vi "Read XML_Extra Checks.vi"(8 "error in (no error)":errorcluster, 11 "Channels In":T1[](array[typedef])) -> (0 "error out":errorcluster, 3 "Channels Out":T1[](array[typedef]))   [LabVIEW 2020]
doc: "This VI performs extra checks (to what is done via the XML Deserializer with the XSD)."
uses:
  XML_Channel.ctl
  XML_Label.ctl
  XML_Parameter.ctl
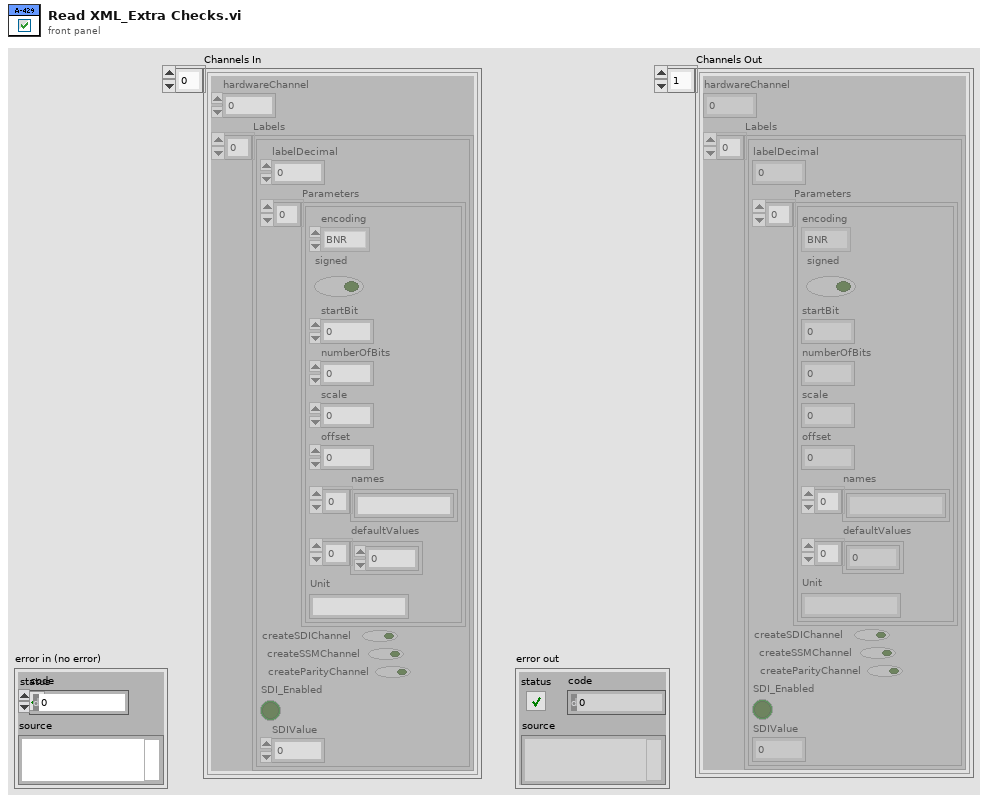
[diagram p1: front panel]
types:
  T1 = typedef "XML_Channel.ctl" = cluster{"hardwareChannel":i32, "Labels":T2[]}
  T2 = typedef "XML_Label.ctl" = cluster{"labelDecimal":i32, "Parameters":T3[], "createSDIChannel":bool, "createSSMChannel":bool, "createParityChannel":bool, "SDI_Enabled":bool, "SDIValue":u8}
  T3 = typedef "XML_Parameter.ctl" = cluster{"encoding":enum16{"BNR", "BCD", "Discrete"}, "signed":bool, "startBit":i32, "numberOfBits":i32, "scale":dbl, "offset":dbl, "names":string[], "defaultValues":dbl[], "Unit":string}
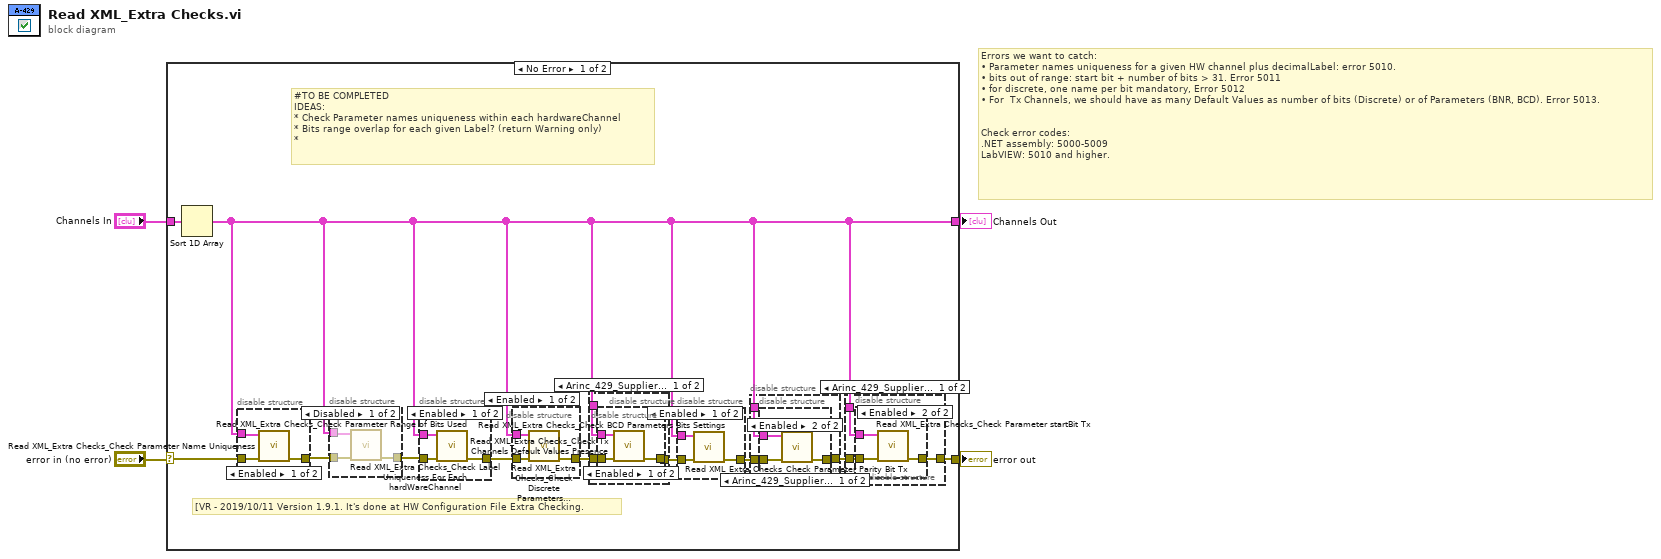
[diagram p0: block diagram]
diagram:
  # "Errors we want to catch:\n•\tParameter names uniqueness for a given HW channel plus decimalLabel: error 5010.\n•\tbits out of range: start bit + number of bits > 31. Error 5011\n•\tfor discrete, one name per bit mandatory, Error 5012\n•\tFor  Tx Channels, we should have as many Default Values as number of bits (Discrete) or of Parameters (BNR, BCD). Error 5013.\n\n\nCheck error codes:\n.NET assembly: 5000-5009\nLabVIEW: 5010 and higher."
  n1 = case shown="No Error" "error in (no error)" {
    selector: "error in (no error)" -> [w14 w61]
    tunnel: [w9 w61] -> w3
    tunnel: "Channels In" -> [w15 w60]
    tunnel: [w6 w60] -> w1
    frame No Error {
      # "[VR - 2019/10/11 Version 1.9.1. It's done at HW Configuration File Extra Checking."
      # "#TO BE COMPLETED\nIDEAS:\n* Check Parameter names uniqueness within each hardwareChannel\n* Bits range overlap for each given Label? (return Warning only)\n*"
      n2 = Sort 1D Array(array=w15) -> (sorted array=w6:T1[])
      n3 = disable-structure shown="Enabled" {
        disable-tunnel: w14 -> [w58 w59]
        disable-tunnel: [w57 w59] -> w7
        disable-tunnel: w6 -> [w56 _]
        frame Enabled {
          n4 = call "Read XML_Extra Checks_Check Parameter Name Uniqueness.vi"("error in (no error)"=w58, "Channels In"=w56) -> ("error out"=w57:errorcluster)  [unwired: 9 in]
        }
        frame Disabled {
        }
      }
      n5 = disable-structure shown="Disabled" {
        disable-tunnel: w7 -> [w18 w19]
        disable-tunnel: [w17 w19] -> w5
        disable-tunnel: w6 -> [w16 _]
        frame Disabled {
          n6 = call "Read XML_Extra Checks_Check Label Uniqueness For Each hardWareChannel.vi"("error in (no error)"=w18, "Channels In"=w16) -> ("error out"=w17:errorcluster)  [unwired: 9 in]
        }
        frame Enabled {
        }
      }
      n7 = disable-structure shown="Enabled" {
        disable-tunnel: w6 -> [w54 _]
        disable-tunnel: w5 -> [w53 w55]
        disable-tunnel: [w52 w55] -> w13
        frame Enabled {
          n8 = call "Read XML_Extra Checks_Check Parameter Range of Bits Used.vi"("error in (no error)"=w53, "Channels In"=w54) -> ("error out"=w52:errorcluster)  [unwired: 9 in]
        }
        frame Disabled {
        }
      }
      n9 = disable-structure shown="Enabled" {
        disable-tunnel: w13 -> [w50 w51]
        disable-tunnel: [w49 w51] -> w12
        disable-tunnel: w6 -> [w48 _]
        frame Enabled {
          n10 = call "Read XML_Extra Checks_Check Discrete Parameters Names.vi"("error in (no error)"=w50, "Channels In"=w48) -> ("error out"=w49:errorcluster)  [unwired: 9 in]
        }
        frame Disabled {
        }
      }
      n11 = disable-structure shown="Arinc_429_Supplier==Ballard, Default" {
        disable-tunnel: w12 -> [w38 w43]
        disable-tunnel: [w37 w43] -> w11
        disable-tunnel: w6 -> [w36 _]
        frame condition #0 (active) {
          n12 = disable-structure shown="Enabled" {
            disable-tunnel: w38 -> [w41 w42]
            disable-tunnel: [w40 w42] -> w37
            disable-tunnel: w36 -> [w39 _]
            frame Enabled {
              n13 = call "Read XML_Extra Checks_Check Tx Channels Default Values Presence.vi"("error in (no error)"=w41, "Channels In"=w39) -> ("error out"=w40:errorcluster)  [unwired: 9 in]
            }
            frame Disabled {
            }
          }
        }
        frame condition #1 {
        }
      }
      n14 = disable-structure shown="Enabled" {
        disable-tunnel: w11 -> [w46 w47]
        disable-tunnel: [w45 w47] -> w10
        disable-tunnel: w6 -> [w44 _]
        frame Enabled {
          n15 = call "Read XML_Extra Checks_Check BCD Parameters Bits Settings.vi"("error in (no error)"=w46, "Channels In"=w44) -> ("error out"=w45:errorcluster)  [unwired: 9 in]
        }
        frame Disabled {
        }
      }
      n16 = disable-structure shown="Arinc_429_Supplier==Ballard, Default" {
        disable-tunnel: w10 -> [w30 w35]
        disable-tunnel: [w29 w35] -> w8
        disable-tunnel: w6 -> [w28 _]
        frame condition #0 (active) {
          n17 = disable-structure shown="Enabled" {
            disable-tunnel: w28 -> [_ w33]
            disable-tunnel: w30 -> [w31 w34]
            disable-tunnel: [w31 w32] -> w29
            frame Disabled {
            }
            frame Enabled {
              n18 = call "Read XML_Extra Checks_Check Parameter Parity Bit Tx.vi"("error in (no error)"=w34, "Channels In"=w33) -> ("error out"=w32:errorcluster)  [unwired: 9 in]
            }
          }
        }
        frame condition #1 {
        }
      }
      n19 = disable-structure shown="Arinc_429_Supplier==Ballard, Default" {
        disable-tunnel: [w22 w27] -> w9
        disable-tunnel: w8 -> [w21 w27]
        disable-tunnel: w6 -> [w20 _]
        frame condition #0 (active) {
          n20 = disable-structure shown="Enabled" {
            disable-tunnel: w20 -> [_ w25]
            disable-tunnel: w21 -> [w23 w26]
            disable-tunnel: [w23 w24] -> w22
            frame Disabled {
            }
            frame Enabled {
              n21 = call "Read XML_Extra Checks_Check Parameter startBit Tx.vi"("error in (no error)"=w26, "Channels In"=w25) -> ("error out"=w24:errorcluster)  [unwired: 9 in]
            }
          }
        }
        frame condition #1 {
        }
      }
    }
    frame Error {
    }
  }
  "error out" <- w3
  "Channels Out" <- w1
